vi "Parse UDP String.vi"(1 "UDP Packet In":string) -> (0 "Array":dbl[][](array[numeric]))   [LabVIEW 2011]
panel:
  in  "Regular Expression":string="[0-9]+\\.[0-9]+"
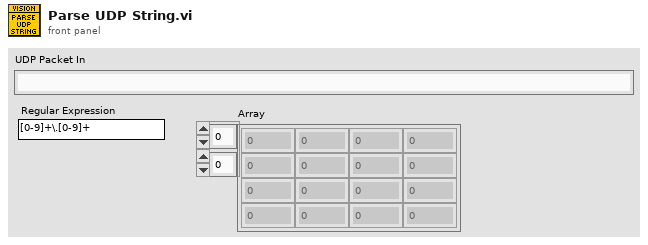
[diagram p1: front panel]
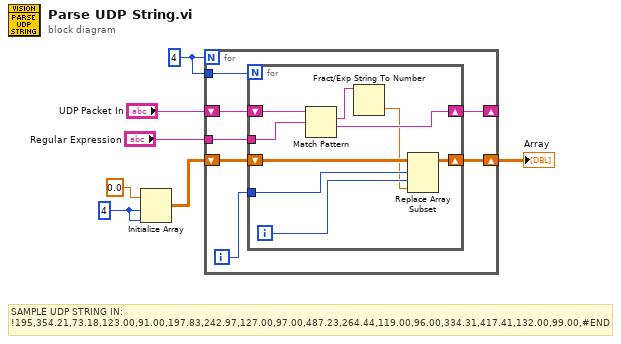
[diagram p0: block diagram]
diagram:
  w4 = 4
  w7 = 4 ("dimension size")
  # "SAMPLE UDP STRING IN:\n!195,354.21,73.18,123.00,91.00,197.83,242.97,127.00,97.00,487.23,264.44,119.00,96.00,334.31,417.41,132.00,99.00,#END"
  n1 = Initialize Array(0.0 ("element"), w7, w7) -> (w2:dbl[][])
  n2 = for {
    N: w4 -> [_]
    shift-right: [w13] -> _
    shift-left: "UDP Packet In" -> [w14]
    tunnel: "Regular Expression" -> [w12]
    tunnel: w4 -> [w11]
    shift-right: [w8] -> w1
    shift-left: w2 -> [w10]
    i -> [w9]
    n3 = for {
      N: w11 -> [_]
      shift-right: [w22] -> w13
      shift-left: w14 -> [w23]
      tunnel: w12 -> [w21]
      tunnel: w9 -> [w19]
      shift-right: [w17] -> w8
      shift-left: w10 -> [w20]
      i -> [w18]
      n4 = Match Pattern(string=w23, regular expression=w21) -> (match substring=w16:string, after substring=w22:string)  [unwired: 1 in, 2 out]
      n5 = Fract/Exp String To Number(string=w16) -> (number=w15:dbl)  [unwired: 3 in, 1 out]
      n6 = Replace Array Subset(array=w20, new element=w15, index (row)=w19, index (col)=w18) -> (w17:dbl[][])
    }
  }
  "Array" <- w1
